vi "Write U64.vi"(8 "error in (no error)":errorcluster, 9 "Data":u64, 10 "Channel Name":string, 11 "CIFCorePlugin in":refnum<class "CIFCorePlugin.lvclass">) -> (0 "error out":errorcluster, 1 "timed out?":bool, 3 "CIFCorePlugin out":refnum<class "CIFCorePlugin.lvclass">)   [LabVIEW 2021, in "CIFCorePlugin.lvclass"]
uses:
  CIFCorePlugin.lvclass
  CIFCorePlugin.lvclass/CIFCorePlugin.ctl
  CIFUtilities/CIFClocks/Typedef/Errors.ctl
  Common/CIFCoreCommon.lvlib
  <vilib>/Utility/miscctls.llb/LVMapReplaceAction.ctl
  CIFUtilities/CIFChannelMng/CIFChannelMng.lvclass
  CIFUtilities/CIFChannels/CIFChannels.lvclass
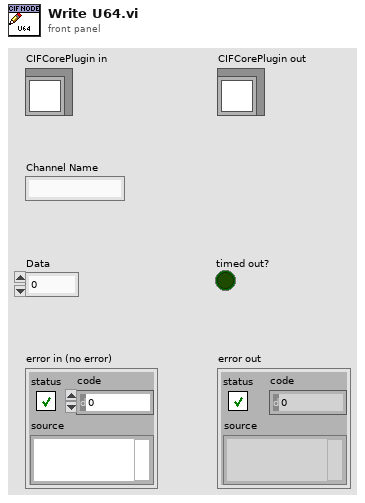
[diagram p1: front panel]
types:
  T1 = typedef "CIFCoreCommon.lvlib/Errors.ctl" = enum16{"Invalid Clock ID", "Long Sleep", "gRPC Server Not Found", "Config Parse", "Timestamp Wrap", "Delayed Execution", "Duplicate Channel", "Missing Channel", "Incorrect Type", "Unregistered Enum"}
  T2 = typedef "LVMapReplaceAction.ctl" = enum32{"Modify Entry only if found", "Add or Modify Entry", "Delete Entry"}
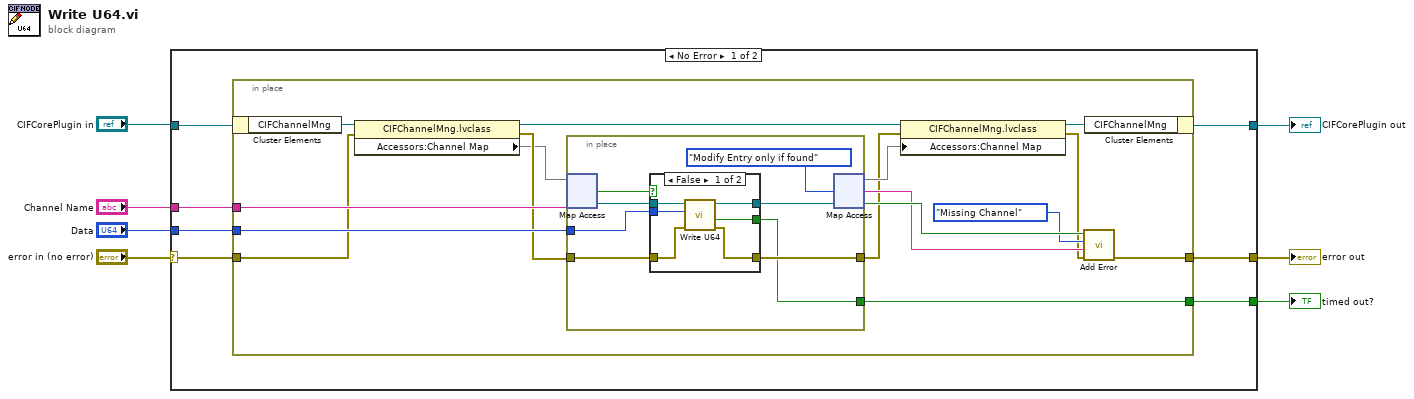
[diagram p0: block diagram]
diagram:
  n1 = case shown="No Error" "error in (no error)" {
    selector: "error in (no error)" -> [w14 w48]
    tunnel: [w12 w48] -> w2
    tunnel: [w8 w47] -> w3
    tunnel: "CIFCorePlugin in" -> [w9 w47]
    tunnel: "Channel Name" -> [w13 _]
    tunnel: "Data" -> [w11 _]
    tunnel: [w10 _] -> w4
    frame No Error {
      n2 = in-place {
        in-place-border: w14 -> [w20]
        in-place-border: w13 -> [w30]
        in-place-border: [w29] -> w12
        in-place-border: w11 -> [w28]
        in-place-border: [w27] -> w10
        n3 = in-place-cluster #1(w9) -> ("CIFChannelMng"=w23:refnum<class "CIFChannelMng.lvclass">)
        n4 = property class="CIFChannelMng.lvclass"(reference=w23, error in=w20) -> (reference out=w22:refnum<class "CIFChannelMng.lvclass">, error out=w19:errorcluster, "Accessors:Channel Map"=w18:map{string, refnum<class "CIFChannels.lvclass">})
        n5 = in-place {
          in-place-border: w19 -> [w35]
          in-place-border: [w34] -> w16
          in-place-border: [w32] -> w27
          in-place-border: w28 -> [w31]
          n6 = in-place-map #2(w18, w30) -> (w37:refnum<class "CIFChannels.lvclass">, w33:bool)  [unwired: 1 in]
          n7 = case shown="False" w33 {
            tunnel: w37 -> [w44 w46]
            tunnel: [w43 w46] -> w36
            tunnel: w35 -> [w42 w45]
            tunnel: [w41 w45] -> w34
            tunnel: [w40 _] -> w32
            tunnel: w31 -> [w39 _]
            frame False {
              n8 = call-dynamic "Write U64.vi"("error in (no error)"=w42, "Data"=w39, "CIFChannels in"=w44) -> ("error out"=w41:errorcluster, "timed out?"=w40:bool, "CIFChannels out"=w43:refnum<class "CIFChannels.lvclass">)  [unwired: 6 in]
            }
            frame True {
            }
          }
          n9 = in-place-map #2(w36, LVMapReplaceAction."Modify Entry only if found" ("action")) -> (w17:map{string, refnum<class "CIFChannels.lvclass">}, w25:string, w26:bool)
        }
        n10 = property class="CIFChannelMng.lvclass"(reference=w22, error in=w16, "Accessors:Channel Map"=w17) -> (reference out=w21:refnum<class "CIFChannelMng.lvclass">, error out=w15:errorcluster)
        n11 = call "Add Error.vi"("error in (no error)"=w15, "String to Append"=w25, "Error"=Errors."Missing Channel", "Insert Error"=w26) -> ("error out"=w29:errorcluster)  [unwired: 7 in]
        n12 = in-place-cluster #1("CIFChannelMng"=w21) -> (w8:refnum<class "CIFCorePlugin.lvclass">)
      }
    }
    frame Error {
    }
  }
  "error out" <- w2
  "CIFCorePlugin out" <- w3
  "timed out?" <- w4
